vi "Exe Version.vi"(11 "Title (Dev only)":string) -> (2 "Version":string, 3 "Title v1.0.0.0":string)   [LabVIEW 2018, in "Main.lvlib"]
uses:
  Main.lvlib
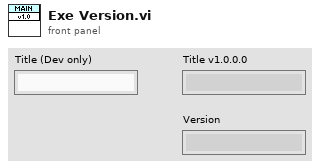
[diagram p1: front panel]
types:
  T1 = enum32{"invalid app kind", "Development System", "Run Time System", "Student Edition", "Embedded LabVIEW", "Evaluation", "Custom"}
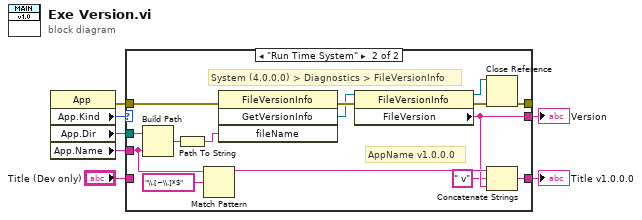
[diagram p0: block diagram]
diagram:
  n1 = property class="App"() -> (error out=w4:errorcluster, "App.Kind"=w5:T1, "App.Dir"=w7:path, "App.Name"=w6:string)  [unwired: 2 in, 1 out]
  n2 = case shown="\"Run Time System\"" w5 {
    tunnel: w7 -> [_ w24]
    tunnel: w6 -> [_ w14]
    tunnel: w4 -> [w8 w22]
    tunnel: [w8 w16] -> _
    tunnel: [_ w12] -> w3
    tunnel: [w9 w10] -> w2
    tunnel: "Title (Dev only)" -> [w9 _]
    frame Default {
    }
    frame "Run Time System" {
      # "AppName v1.0.0.0"
      # "System (4.0.0.0) > Diagnostics > FileVersionInfo"
      n3 = Build Path(base path=w24, name or relative path=w14) -> (appended path=w23:path)
      n4 = Path To String(path=w23) -> (string=w21:string)
      n5 = Match Pattern(string=w14, regular expression="\\.[~\\.]*$") -> (before substring=w13:string)  [unwired: 4 out]
      n6 = invoke class="FileVersionInfo" method="GetVersionInfo"(error in=w22, "fileName"=w21) -> (error out=w20:errorcluster, "GetVersionInfo"=w19:refnum<k24>)  [unwired: 2 in, 2 out]
      n7 = property class="FileVersionInfo"(reference=w19, error in=w20) -> (reference out=w17:refnum<k24>, error out=w18:errorcluster, "FileVersion"=w12:string)
      n8 = Close Reference(reference=w17, error in (no error)=w18) -> (error out=w16:errorcluster)
      n9 = Concatenate Strings(w13, " v" ("string"), w12) -> (w10:string)
    }
  }
  "Title v1.0.0.0" <- w2
  "Version" <- w3
